vi "CameraVision.vi"(0 "X2 Change":dbl, 1 "X1 Change":dbl, 4 "W":dbl=20.22, 6 "Distance Change":dbl=-7.0, 7 "x2":dbl, 8 "x":dbl, 9 "Left FOV":dbl=35.735, 10 "Right FOV":dbl=34.727) -> (2 "Angle to Target":dbl, 3 "Distance to Target":dbl)   [LabVIEW 2013]
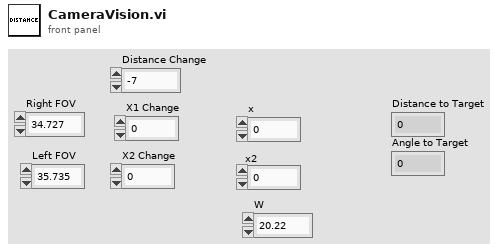
[diagram p1: front panel]
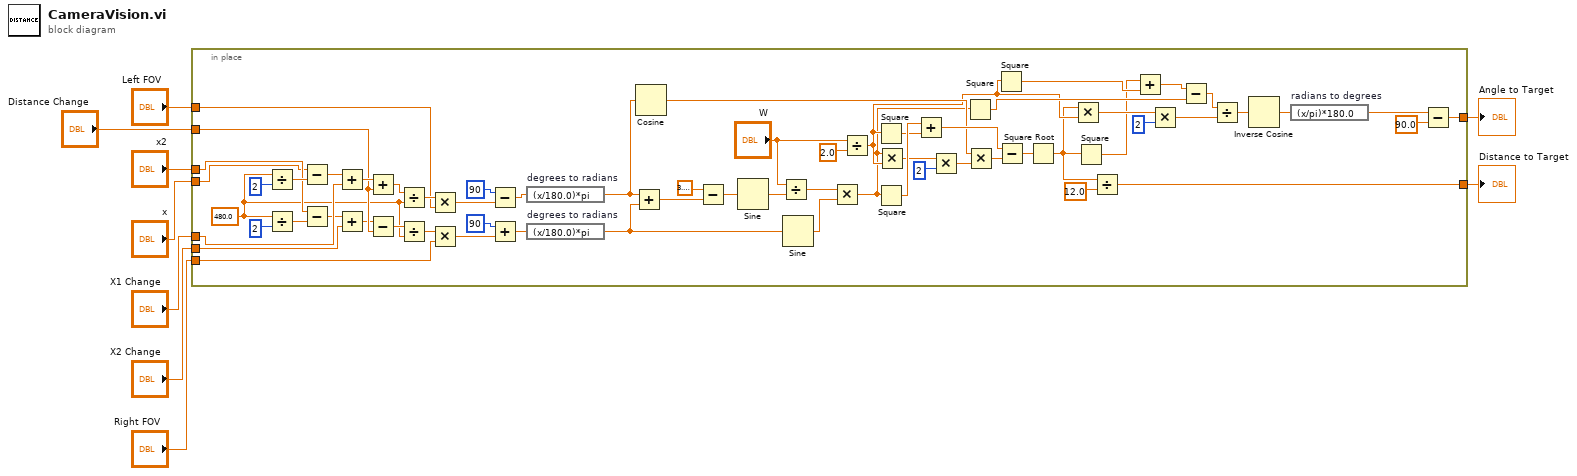
[diagram p0: block diagram]
diagram:
  n1 = in-place {
    in-place-border: "x2" -> [w66]
    in-place-border: "x" -> [w65]
    in-place-border: "X1 Change" -> [w60]
    in-place-border: "X2 Change" -> [w59]
    in-place-border: [w56] -> w5
    in-place-border: [w54] -> w4
    in-place-border: "Distance Change" -> [w52]
    in-place-border: "Right FOV" -> [w45]
    in-place-border: "Left FOV" -> [w44]
    w46 = 480.0 ("y")
    n2 = Divide(x=w46, y=2) -> (x/y=w67:dbl)
    n3 = Divide(x=w46, y=2) -> (x/y=w70:dbl)
    n4 = Subtract(x=w65, y=w67) -> (x-y=w48:dbl)
    n5 = Subtract(x=w66, y=w70) -> (x-y=w51:dbl)
    n6 = Add(x=w48, y=w60) -> (x+y=w53:dbl)
    n7 = Add(x=w51, y=w59) -> (x+y=w50:dbl)
    n8 = Add(x=w53, y=w52) -> (x+y=w47:dbl)
    n9 = Subtract(x=w50, y=w52) -> (x-y=w49:dbl)
    n10 = Divide(x=w47, y=w46) -> (x/y=w71:dbl)
    n11 = Divide(x=w49, y=w46) -> (x/y=w72:dbl)
    n12 = Multiply(x=w71, y=w44) -> (x*y=w62:dbl)
    n13 = Multiply(x=w72, y=w45) -> (x*y=w61:dbl)
    n14 = Subtract(x=90, y=w62) -> (x-y=w16:dbl)
    n15 = Add(x=90, y=w61) -> (x+y=w14:dbl)
    n16 = expression code="(x/180.0)*pi" "degrees to radians"(w16) -> (w15:dbl)
    n17 = expression code="(x/180.0)*pi" "degrees to radians"(w14) -> (w13:dbl)
    n18 = Add(x=w15, y=w13) -> (x+y=w43:dbl)
    n19 = Cosine(x=w15) -> (cos(x)=w30:dbl)
    n20 = Subtract(x=3.141592653589793, y=w43) -> (x-y=w41:dbl)
    n21 = Sine(x=w41) -> (sin(x)=w40:dbl)
    n22 = Divide(x="W", y=w40) -> (x/y=w39:dbl)
    n23 = Sine(x=w13) -> (sin(x)=w38:dbl)
    n24 = Multiply(x=w39, y=w38) -> (x*y=w19:dbl)
    n25 = Divide(x="W", y=2.0) -> (x/y=w20:dbl)
    n26 = Square(x=w20) -> (x^2=w35:dbl)
    n27 = Square(x=w19) -> (x^2=w36:dbl)
    n28 = Multiply(x=w19, y=w20) -> (x*y=w32:dbl)
    n29 = Add(x=w36, y=w35) -> (x+y=w34:dbl)
    n30 = Multiply(x=w32, y=2) -> (x*y=w31:dbl)
    n31 = Square(x=w19) -> (x^2=w22:dbl)
    n32 = Multiply(x=w30, y=w31) -> (x*y=w29:dbl)
    n33 = Square(x=w20) -> (x^2=w23:dbl)
    n34 = Subtract(x=w34, y=w29) -> (x-y=w12:dbl)
    n35 = Square Root(x=w12) -> (sqrt(x)=w11:dbl)
    n36 = Multiply(x=w11, y=w20) -> (x*y=w27:dbl)
    n37 = Square(x=w11) -> (x^2=w10:dbl)
    n38 = Divide(x=w11, y=12.0) -> (x/y=w54:dbl)
    n39 = Add(x=w10, y=w23) -> (x+y=w28:dbl)
    n40 = Multiply(x=w27, y=2) -> (x*y=w24:dbl)
    n41 = Subtract(x=w28, y=w22) -> (x-y=w25:dbl)
    n42 = Divide(x=w25, y=w24) -> (x/y=w21:dbl)
    n43 = Inverse Cosine(1:w21) -> (0:w18:dbl)
    n44 = expression code="(x/pi)*180.0" "radians to degrees"(w18) -> (w17:dbl)
    n45 = Subtract(x=w17, y=90.0) -> (x-y=w56:dbl)
  }
  "Distance to Target" <- w4
  "Angle to Target" <- w5
